vi "deney_8_5.vi"() -> ()   [LabVIEW 2018]
panel:
  in  "cevaplar":string[](array[string])
  out "SAYI":u16
  in  "Tahmin":u16
  out "BITTI":bool
  out "KALAN":i32=10
  out "MESAJ":string="Tahmin : 0 .. 1023"
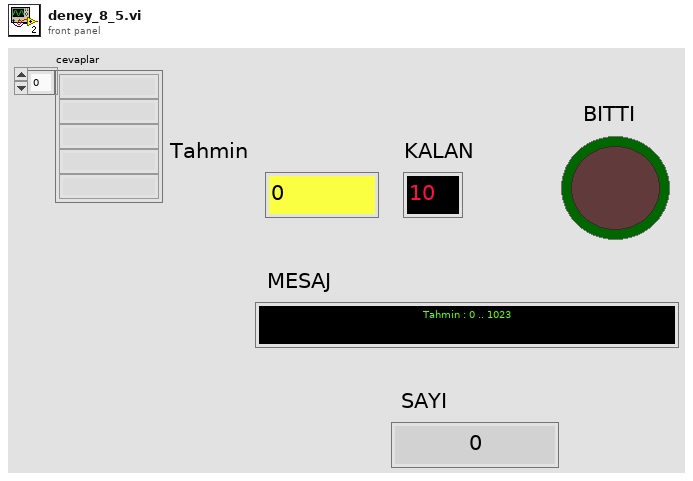
[diagram p1: front panel]
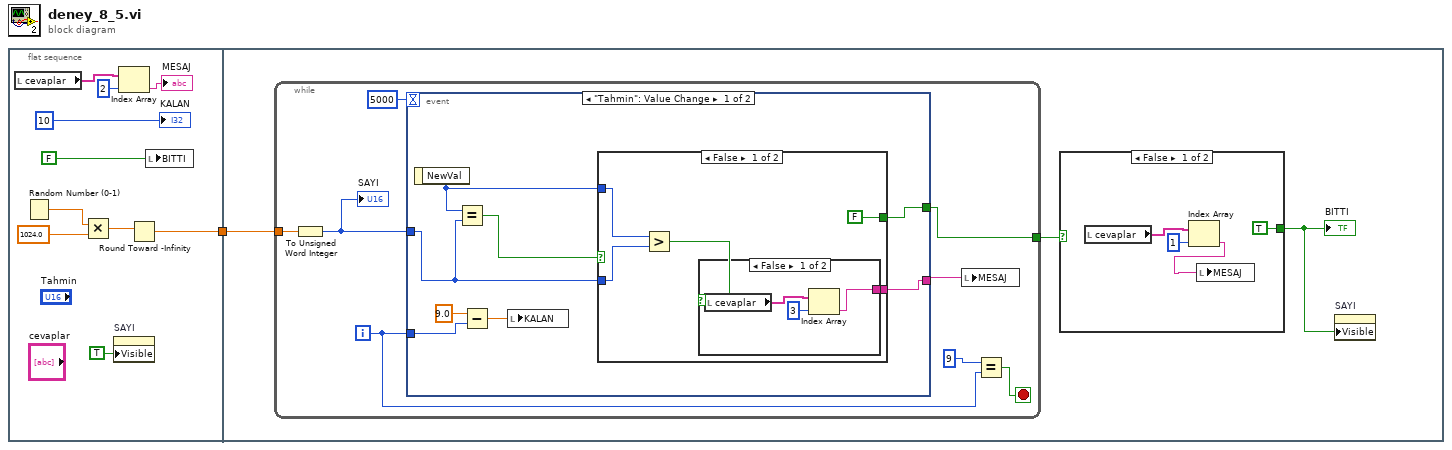
[diagram p0: block diagram]
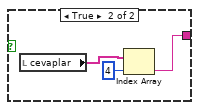
[diagram p2: hidden frame]
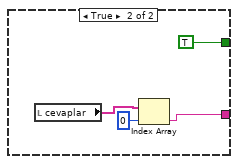
[diagram p3: hidden frame]
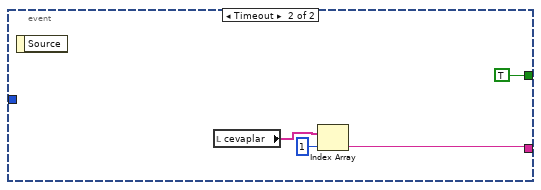
[diagram p4: hidden frame]
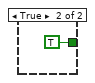
[diagram p5: hidden frame]
diagram:
  n1 = flat-sequence {
    tunnel: [w7] -> w1
    tunnel: w1 -> [w14]
    frame #0 {
      n2 = local read "cevaplar"() -> (w4:string[])
      n3 = Random Number (0-1)() -> (number: 0 to 1=w9:dbl)
      n4 = Multiply(x=w9, y=1024.0) -> (x*y=w8:dbl)
      n5 = property on="SAYI" class="DigNum (strict)"("Visible"=TRUE) -> ()  [unwired: 2 in, 2 out]
      n6 = Index Array(array=w4, index=2) -> (element=→"MESAJ":string)
      n7 = Round Toward -Infinity(1:w8) -> (0:w7:dbl)
      n8 = local write "BITTI"(FALSE ("BITTI")) -> ()
      "KALAN" <- 10
    }
    frame #1 {
      n9 = while {
        tunnel: w14 -> [w22]
        tunnel: [w19] -> w13
        i -> [w16]
        stop <- w15 stop-if-true
        n10 = To Unsigned Word Integer(number=w22) -> (unsigned 16bit integer=w21:u16)
        "SAYI" <- w21
        n11 = event shown="[0] \"Tahmin\": Value Change" {
          selector: _ -> [_ _]
          dyn-events: _ -> [_ _]
          timeout: 5000 -> [_ _]
          tunnel: w21 -> [w30 _]
          tunnel: w16 -> [w27 _]
          tunnel: [w24 TRUE] -> w19
          tunnel: [w23 w46] -> w20
          event "Tahmin": Value Change {
            n12 = event-data() -> ("NewVal"=w25:u16)  [unwired: 1 in]
            n13 = Equal?(x=w25, y=w30) -> (x = y?=w29:bool)
            n14 = Subtract(x=9.0, y=w27) -> (x-y=w26:dbl)
            n15 = local write "KALAN"(w26) -> ()
            n16 = case shown="False" w29 {
              tunnel: w30 -> [w34 _]
              tunnel: w25 -> [w35 _]
              tunnel: [FALSE TRUE] -> w24
              tunnel: [w32 w42] -> w23
              frame False {
                n17 = Greater?(x=w35, y=w34) -> (0:w33:bool)
                n18 = case shown="False" w33 {
                  tunnel: [w36 w39] -> w32
                  frame False {
                    n19 = local read "cevaplar"() -> (w37:string[])
                    n20 = Index Array(array=w37, index=3) -> (element=w36:string)
                  }
                  frame True {
                    n21 = local read "cevaplar"() -> (w41:string[])
                    n22 = Index Array(array=w41, index=4) -> (element=w39:string)
                  }
                }
              }
              frame True {
                n23 = local read "cevaplar"() -> (w44:string[])
                n24 = Index Array(array=w44, index=0) -> (element=w42:string)
              }
            }
          }
          event Timeout {
            n25 = event-data() -> ()  [unwired: 1 in, 1 out]
            n26 = local read "cevaplar"() -> (w47:string[])
            n27 = Index Array(array=w47, index=1) -> (element=w46:string)
          }
        }
        n28 = local write "MESAJ"(w20) -> ()
        n29 = Equal?(x=9, y=w16) -> (x = y?=w15:bool)
      }
      n30 = case shown="False" w13 {
        tunnel: [TRUE TRUE] -> w12
        frame False {
          n31 = local read "cevaplar"() -> (w52:string[])
          n32 = Index Array(array=w52, index=1) -> (element=w50:string)
          n33 = local write "MESAJ"(w50) -> ()
        }
        frame True {
        }
      }
      "BITTI" <- w12
      n34 = property on="SAYI" class="DigNum (strict)"("Visible"=w12) -> ()  [unwired: 2 in, 2 out]
    }
  }
